vi "Array of I64_Read Index.vi"(9 "Default":i64[](array[numeric]), 11 "Index":i32) -> (1 "Value":i64[](array[numeric]))   [LabVIEW 2010, in "Current Value Table.lvlib"]
doc: "This VI takes a memory index (I32) and will perform a read on that index. This VI will never return the default value, as it has no error handling for increased performance. If the index is invalid, the default for the data type will be returned."
uses:
  Current Value Table.lvlib
  Type Defs/Memory Commands.ctl
  Array of I64_Memory Block.vi
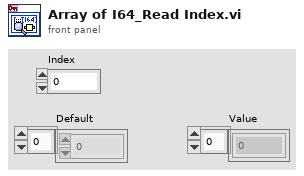
[diagram p1: front panel]
types:
  T1 = typedef "Current Value Table.lvlib/Memory Commands.ctl" = enum16{"Init", "Add Data", "Read", "Read Group", "Read All", "Write", "Write Group", "Get Size"}
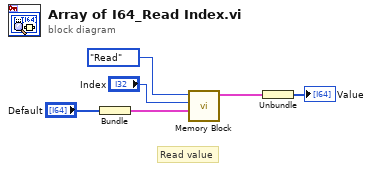
[diagram p0: block diagram]
diagram:
  # "Read value"
  n1 = Bundle("Default"="Default") -> (w4:cluster{"Default":i64[]})  [unwired: 1 in]
  n2 = call-poly "Memory Block.vi"("Value"=w4, "Index"="Index", "Method"=Memory_Commands."Read") -> ("Value Out"=w2:cluster{"I64 Array":i64[]})  [unwired: 6 in, 2 out]
  n3 = Unbundle(w2) -> ("I64 Array"=→"Value":i64[])
